vi "PalmSense Action-Status.vi"(8 "error in (no error)":errorcluster, 10 "Message Data":variant, 11 "Data Cluster":T1) -> (0 "error out":errorcluster, 3 "Data Cluster out":T1)   [LabVIEW 2020, in "PalmSens.lvlib"]
uses:
  PalmSens.lvlib
  PalmSense Hardware Configuration.ctl
  <instrlib>/PalmSens SDK for LabVIEW 5.10/PalmSens/PalmSens.lvclass
  support/Message Queue/Message Cluster.ctl
  support/Message Queue/Message Queue.lvlib
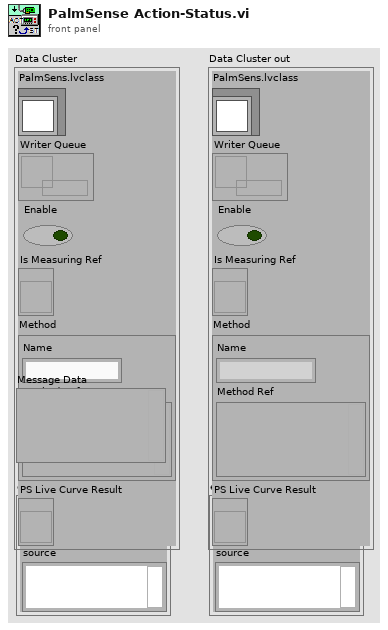
[diagram p1: front panel]
types:
  T1 = typedef "PalmSens.lvlib/PalmSense Hardware Configuration.ctl" = cluster{"PalmSens.lvclass":refnum<class "PalmSens.lvclass">, "Writer Queue":refnum<queue>, "Enable":bool, "Is Measuring Ref":refnum<vi>, "Method":cluster{"Name":string, "Method Ref":variant}, "PS Live Curve Result":refnum<vi>}
  T2 = typedef "Message Queue.lvlib/Message Cluster.ctl" = cluster{"Message":string, "Message Data":variant}
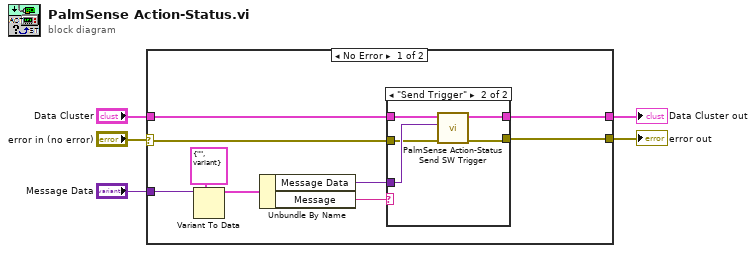
[diagram p0: block diagram]
diagram:
  n1 = case shown="No Error" "error in (no error)" {
    selector: "error in (no error)" -> [w9 w22]
    tunnel: [w14 w22] -> w5
    tunnel: "Data Cluster" -> [w7 w23]
    tunnel: [w6 w23] -> w3
    tunnel: "Message Data" -> [w10 _]
    frame No Error {
      n2 = Variant To Data(type=T2 {"Message"="", "Message Data"=variant} ("element"), Variant=w10) -> (data=w12:T2)  [unwired: 1 in, 1 out]
      n3 = Unbundle By Name(w12) -> ("Message Data"=w8:variant, "Message"=w13:string)
      n4 = case shown="\"Send Trigger\"" w13 {
        tunnel: w8 -> [_ w18]
        tunnel: [w16 w19] -> w6
        tunnel: w7 -> [w16 w20]
        tunnel: w9 -> [w15 w17]
        tunnel: [w15 w21] -> w14
        frame "False", Default {
        }
        frame "Send Trigger" {
          n5 = call "PalmSense Action-Status Send SW Trigger.vi"("error in (no error)"=w17, "Message Data"=w18, "Data Cluster in"=w20) -> ("error out"=w21:errorcluster, "Data Cluster out"=w19:T1)  [unwired: 7 in]
        }
      }
    }
    frame Error {
    }
  }
  "error out" <- w5
  "Data Cluster out" <- w3
